vi "Mini Table Pop Up.vi"(8 "error in (no error)":errorcluster, 10 "Data[][]":string[][](array[string]), 11 "Headers[]":string[](array[string])) -> (0 "error out":errorcluster)   [LabVIEW 2014, in "CSV Analyzer.lvlib"]
uses:
  CSV Analyzer.lvlib
panel:
  in  "Multicolumn Listbox":i32(listbox)
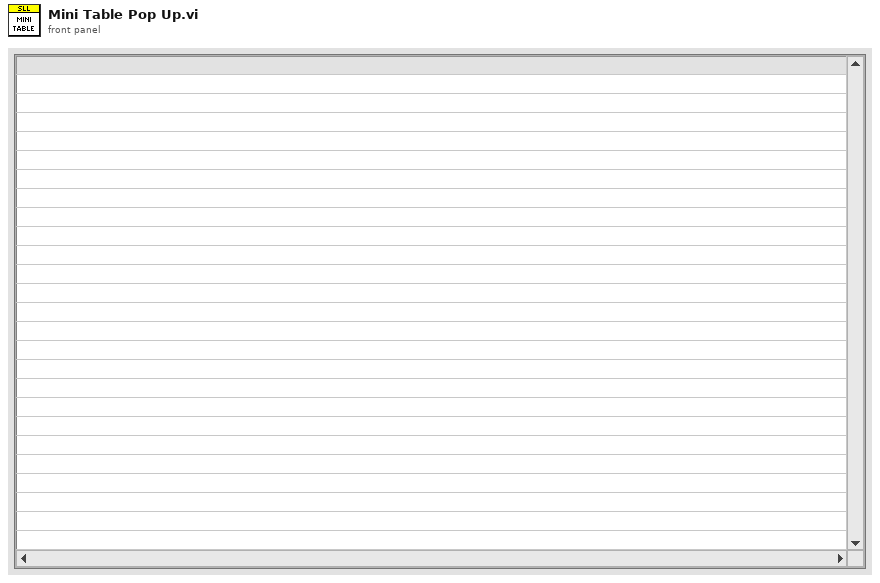
[diagram p1: front panel]
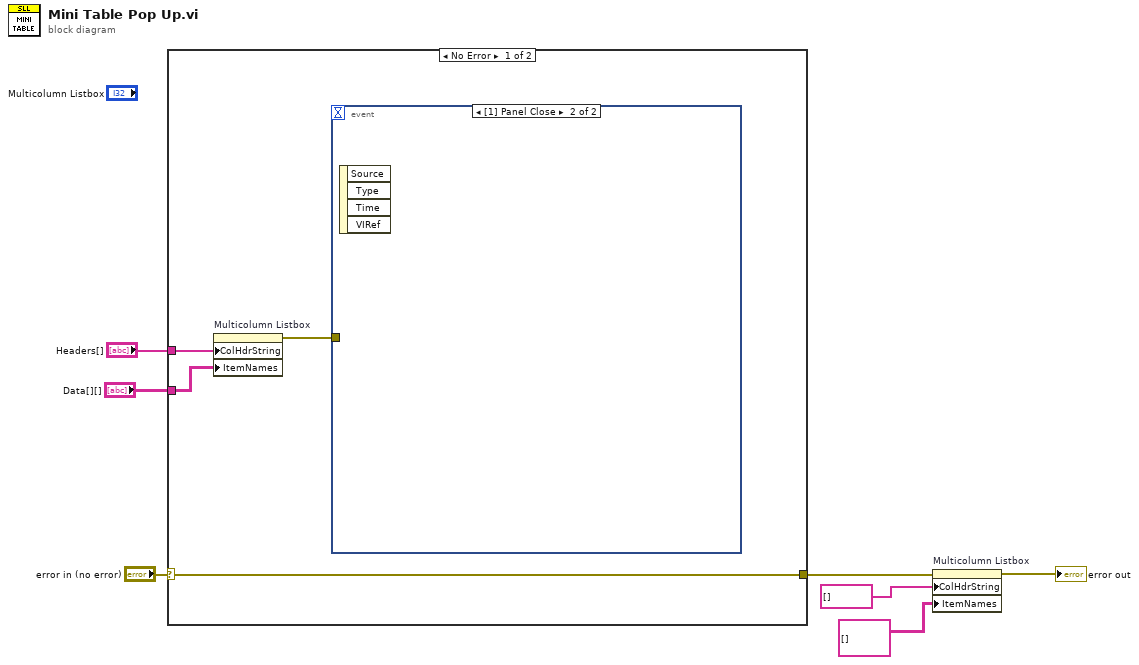
[diagram p0: block diagram]
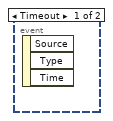
[diagram p2: hidden frame]
diagram:
  n1 = case shown="No Error" "error in (no error)" {
    selector: "error in (no error)" -> [w11 w12]
    tunnel: [w11 w12] -> w4
    tunnel: "Headers[]" -> [w10 _]
    tunnel: "Data[][]" -> [w9 _]
    frame No Error {
      n2 = property on="Multicolumn Listbox" class="MCListbox (strict)"("ColHdrString"=w10, "ItemNames"=w9) -> (error out=w8:errorcluster)  [unwired: 2 in, 1 out]
      n3 = event shown="[1] Panel Close" {
        selector: _ -> [_ _]
        dyn-events: _ -> [_ _]
        timeout: _ -> [_ _]
        tunnel: w8 -> [_ _]
        event Timeout {
          n4 = event-data() -> ()  [unwired: 1 in, 3 out]
        }
        event Panel Close {
          n5 = event-data() -> ()  [unwired: 1 in, 4 out]
        }
      }
    }
    frame Error {
    }
  }
  n6 = property on="Multicolumn Listbox" class="MCListbox (strict)"(error in=w4, "ColHdrString"=string[] [] ("Column Header Strings[]"), "ItemNames"=string[][] [] ("Item Names")) -> (error out=→"error out":errorcluster)  [unwired: 1 in, 1 out]
